vi "F Dwf Digital IO Output Enable Info64.vi"(8 "error in (no error)":errorcluster, 10 "pfsOutputEnableMask":cluster{}, 11 "hdwf":i32) -> (0 "error out":errorcluster, 2 "pfsOutputEnableMask out":cluster{}, 3 "function return":i32)   [LabVIEW 2021, in "Olasdwf.lvlib"]
doc: "DWFAPI int FDwfDigitalIOOutputEnableInfo64(HDWF hdwf, unsigned long long *pfsOutputEnableMask);"
uses:
  Olasdwf.lvlib
  Windows/System32/dwf.dll
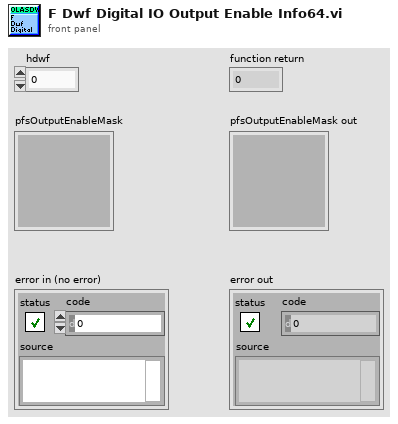
[diagram p1: front panel]
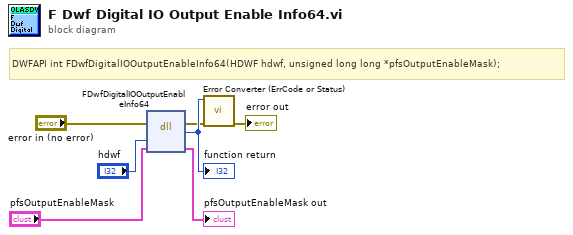
[diagram p0: block diagram]
diagram:
  # "DWFAPI int FDwfDigitalIOOutputEnableInfo64(HDWF hdwf, unsigned long long *pfsOutputEnableMask);"
  n1 = dll-call lib="/Windows/System32/dwf.*" fn="FDwfDigitalIOOutputEnableInfo64"(error in="error in (no error)", "hdwf"="hdwf", "pfsOutputEnableMask"="pfsOutputEnableMask") -> (error out=w2:errorcluster, w7:i32, "pfsOutputEnableMask"=→"pfsOutputEnableMask out":cluster{})  [unwired: 3 in, 1 out]
  "function return" <- w7
  n2 = call "Error Converter (ErrCode or Status).vi"("error in (no error)"=w2, "error code"=w7) -> ("error out"=→"error out":errorcluster)  [unwired: 9 in]
